vi "parse_packet.vi"(11 "Packet In":u8[](array[numeric])) -> (2 "op-code":u16, 3 "Packet Out":u8[](array[numeric]))   [LabVIEW 2024]
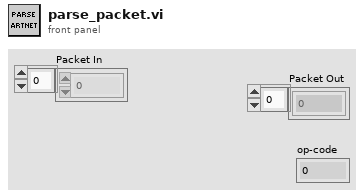
[diagram p1: front panel]
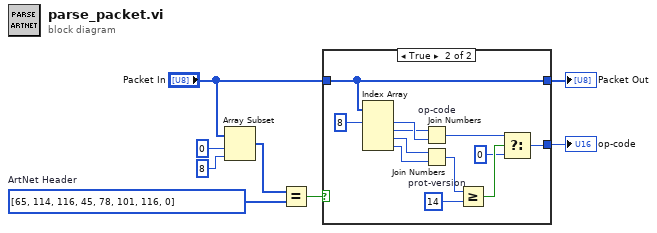
[diagram p0: block diagram]
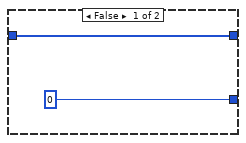
[diagram p2: hidden frame]
diagram:
  w6 = u8[] [65, 114, 116, 45, 78, 101, 116, 0]  # ArtNet Header
  n1 = Array Subset(array="Packet In", index=0, length=8 ("Länge")) -> (w5:u8[])
  n2 = Equal?(x=w5, y=w6) -> (x = y?=w3:bool)
  n3 = case shown="True" w3 {
    tunnel: "Packet In" -> [w10 w15]
    tunnel: [w10 w15] -> w2
    tunnel: [u16 0 w12] -> w1
    frame False {
    }
    frame True {
      n4 = Index Array(array=w15, index #1=8 ("index")) -> (element #1=w21:u8, element #2=w20:u8, element #3=w19:u8, element #4=w18:u8)  [unwired: 3 in]
      n5 = Join Numbers "op-code"(hi=w20, lo=w21) -> ((hi.lo)=w13:u16)
      n6 = Join Numbers "prot-version"(hi=w19, lo=w18) -> ((hi.lo)=w17:u16)
      n7 = Greater Or Equal?(x=w17, y=u16 14) -> (x >= y?=w14:bool)
      n8 = Select(t=w13, s=w14, f=u16 0) -> (s? t:f=w12:u16)
    }
  }
  "Packet Out" <- w2
  "op-code" <- w1
